vi "get configuration by UID.vi"(8 "error in":errorcluster, 10 "UID":string, 11 "CEF_HierarchyRepo in":refnum<class "CEF_HierarchyRepo.lvclass">) -> (0 "error out":errorcluster, 1 "configuration":refnum<class "CEF_serializable configuration.lvclass">, 3 "CEF_HierarchyRepo out":refnum<class "CEF_HierarchyRepo.lvclass">)   [LabVIEW 2025, in "CEF.lvlib" / "CEF_HierarchyRepo.lvclass"]
doc: "Copyright 2017 National Instruments Corporation\n\nLicensed under the Apache License, Version 2.0 (the \"License\"); you may not use this file except in compliance with the License. You may obtain a copy of the License at http://www.apache.org/licenses/LICENSE-2.0\nUnless required by applicable law or agreed to in writing, software distributed under the License is distributed on an \"AS IS\" BASIS, WITHOUT WARRANTIES OR CONDITIONS OF ANY KIND, either express or implied. See the License for the specific language governing permissions and limitations under the License."
uses:
  CEF_HierarchyRepo.lvclass
  serializable configuration/CEF_serializable configuration.lvclass
  CEF_HierarchyRepo.lvclass/CEF_HierarchyRepo.ctl
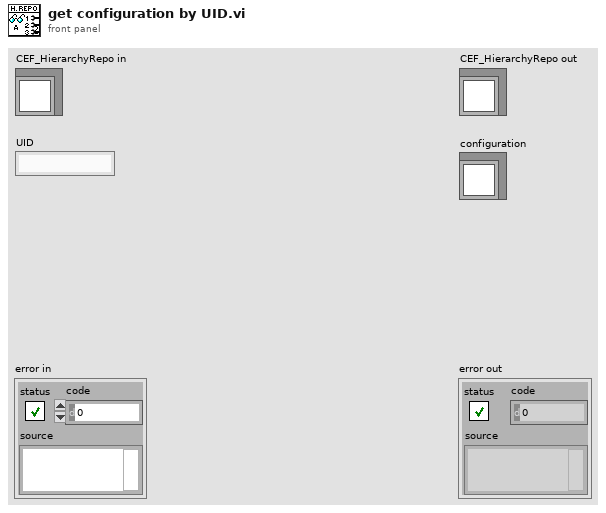
[diagram p1: front panel]
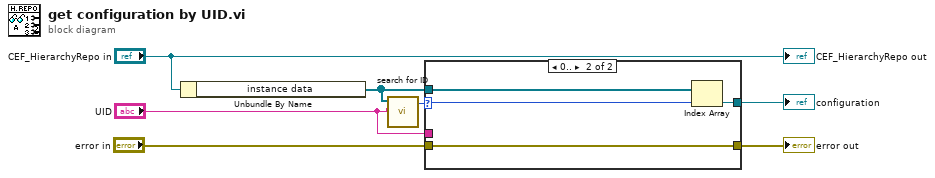
[diagram p0: block diagram]
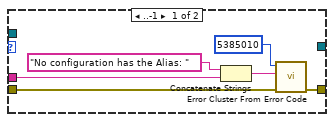
[diagram p2: hidden frame]
diagram:
  n1 = Unbundle By Name("CEF_HierarchyRepo in") -> ("instance data"=w1:refnum<class "CEF_serializable configuration.lvclass">[])
  n2 = call "search for ID.vi"("instance id"="UID", "instance data"=w1) -> ("index"=w2:i32)  [unwired: 9 in]
  n3 = case shown="0.." w2 {
    selector: w2 -> [_ w14]
    tunnel: w1 -> [_ w17]
    tunnel: [_ w16] -> w3
    tunnel: "error in" -> [w13 w15]
    tunnel: [w12 w15] -> w6
    tunnel: "UID" -> [w9 _]
    frame ..-1 {
      n4 = Concatenate Strings("No configuration has the Alias: " ("string"), w9) -> (w10:string)
      n5 = call <vilib>:"Error Cluster From Error Code.vi"("error in (no error)"=w13, "error message (\"\")"=w10, "error code (0)"=5385010) -> ("error out"=w12:errorcluster)  [unwired: 6 in]
    }
    frame 0.. {
      n6 = Index Array(array=w17, index=w14) -> (element=w16:refnum<class "CEF_serializable configuration.lvclass">)
    }
  }
  "error out" <- w6
  "configuration" <- w3
  "CEF_HierarchyRepo out" <- "CEF_HierarchyRepo in"
